vi "MHL_open tdms file.vi"(0 "TDMS_DataHandler in":refnum<class "TDMS_DataHandler.lvclass">, 1 "Message Data":variant, 5 "error in (no error)":errorcluster) -> (14 "TDMS_DataHandler out":refnum<class "TDMS_DataHandler.lvclass">, 19 "error out":errorcluster)   [LabVIEW 2019, in "FileReader.lvlib"]
uses:
  FileReader.lvlib
  Class Library/TDMS_DataHandler_class/TDMS_DataHandler.lvclass
  Open TDMS file Argument--cluster.ctl
  Open TDMS file (Reply Payload)--cluster.ctl
  Class Library/TDMS_DataHandler_class/Fcurve Meta data.ctl
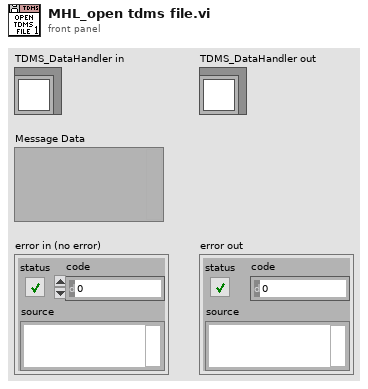
[diagram p1: front panel]
types:
  T1 = typedef "FileReader.lvlib/Open TDMS file (Reply Payload)--cluster.ctl" = cluster{"Group metadata":T2, "Channel name(s)":string[], "Channel datum out":waveform(dbl)[], "size (in bytes)":i64, "error":errorcluster}
  T2 = typedef "TDMS_DataHandler.lvclass/Fcurve Meta data.ctl" = cluster{"property names":string[], "property values":variant[]}
  T3 = typedef "FileReader.lvlib/Open TDMS file Argument--cluster.ctl" = cluster{"Wait Notifier":refnum<notifier>, "wait for reply":bool, "TDMS filepath":path}
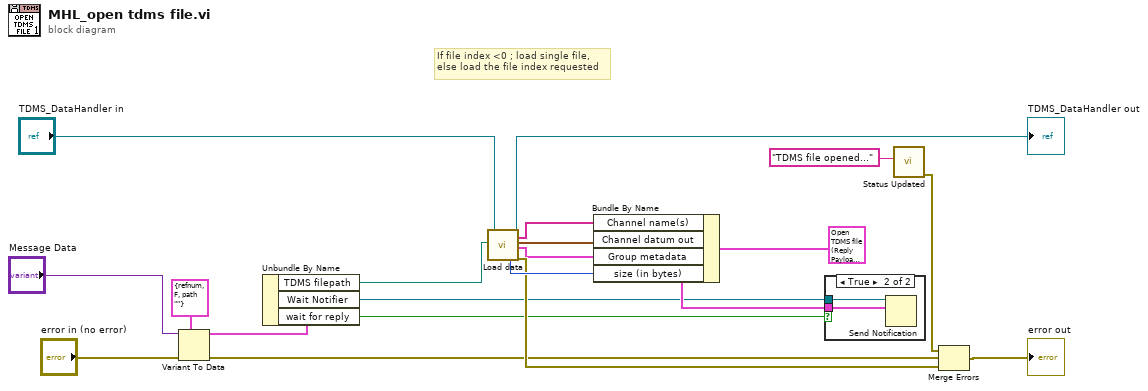
[diagram p0: block diagram]
diagram:
  # "If file index <0 ; load single file,\nelse load the file index requested"
  n1 = Variant To Data(error in="error in (no error)", type=T3 {"Wait Notifier"=refnum, "wait for reply"=FALSE, "TDMS filepath"=path ""} ("Initialize File Argument"), Variant="Message Data") -> (data=w5:T3, error out=w17:errorcluster)
  n2 = Unbundle By Name(w5) -> ("TDMS filepath"=w1:path, "Wait Notifier"=w6:refnum<notifier>, "wait for reply"=w7:bool)
  n3 = call-dynamic "Load data.vi"("reference in"="TDMS_DataHandler in", "TDMS Filepath"=w1) -> ("size (in bytes)"=w20:i64, "reference out"=→"TDMS_DataHandler out":refnum<class "TDMS_DataHandler.lvclass">, "Channel name(s)"=w13:string[], "Channels out"=w11:waveform(dbl)[], "Group metadata"=w12:T2, "error out"=w18:errorcluster)  [unwired: 12 in]
  n4 = Bundle By Name(cluster=T1 {"Group metadata"={"property names"=[], "property values"=[]}, "Channel name(s)"=[], "Channel datum out"=[], "size (in bytes)"=37399506, "error"={"status"=FALSE, "code"=0, "source"=""}} ("Initialize File (Reply Payload)"), "Channel name(s)"=w13, "Channel datum out"=w11, "Group metadata"=w12, "size (in bytes)"=w20) -> (w9:T1)
  n5 = case shown="True" w7 {
    tunnel: w6 -> [_ w22]
    tunnel: w9 -> [_ w21]
    frame False {
    }
    frame True {
      n6 = Send Notification(notification=w21, notifier=w22) -> ()  [unwired: 1 in, 2 out]
    }
  }
  n7 = call "Status Updated.vi"("Status"="TDMS file opened...") -> ("error out"=w19:errorcluster)  [unwired: 10 in]
  n8 = Merge Errors(w19, w17, w18) -> (→"error out":errorcluster)
